vi "demandsView.vi"(10 "UserEvents in":refnum<class "UserEvents.lvclass">) -> ()   [LabVIEW 2013, in "AITDTViews.lvlib"]
uses:
  AITDTViews.lvlib
  UserEvents/UserEvents.lvclass
  CommandFactory/CommandFactory.lvclass
  UserEvents/UserEvents.lvclass/UserEvents.ctl
  Typedefs/StateSelector.ctl
  Typedefs/CommandSelector.ctl
  Typedefs/AITDTTypedefs.lvlib
  ConfigurationTestParameters/ConfigurationTestParameters.lvclass
panel:
  in  "stopTestIsTrue":bool
  in  "startTestIsTrue":bool
types:
  T1 = enum8{"Enabled", "Disabled", "Disabled and Grayed Out"}
  T2 = typedef "AITDTTypedefs.lvlib/PubDataEvents.ctl" = cluster{"State":refnum<user-event>, "ErrorCode":refnum<user-event>, "OutputData":refnum<user-event>, "InputData":refnum<user-event>, "TestStatus":refnum<user-event>, "LogPath":refnum<user-event>, "TemperatureSetpointRequest":refnum<user-event>, "TemperatureSettling":refnum<user-event>, "WaitTimeStatus":refnum<user-event>}
  T3 = typedef "AITDTTypedefs.lvlib/SubDataEvents.ctl" = cluster{"Command":refnum<user-event>}
  T4 = cluster{"Event Registration Refnum":refnum<event-registration>}
  T5 = typedef "AITDTTypedefs.lvlib/StateSelector.ctl" = enum16{"AwaitingSetpointAcknowledgmentState", "EndingCycleState", "FaultState", "OffState", "PausingState", "RequestingNewSetpointState", "SamplingState", "SettlingState", "SoakingState", "StabilizingState", "StandbyState", "StoppedState", "TransitioningTemperatureState"}
  T6 = typedef "AITDTTypedefs.lvlib/CommandSelector.ctl" = enum16{"ClearError", "ConfirmSetpointApplied", "Exit", "StandBy", "Start", "StartTest", "StopTest", "Update"}
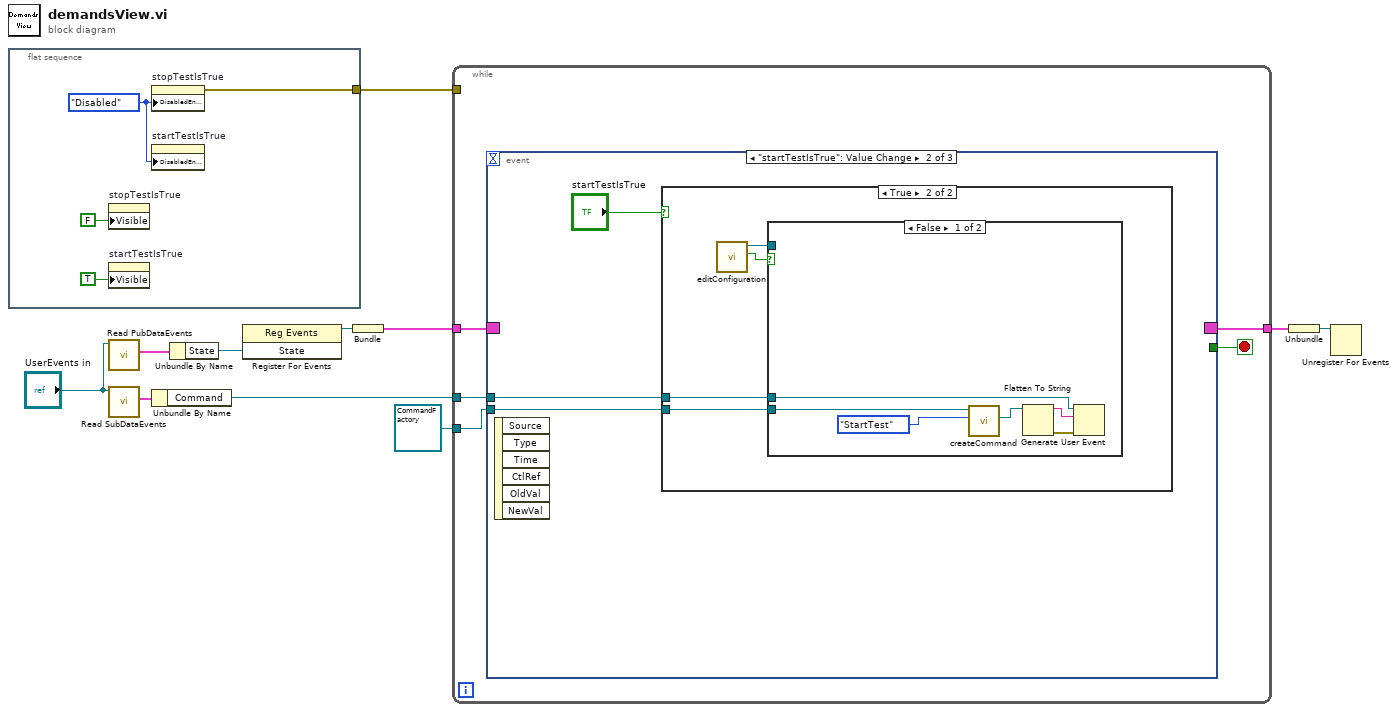
[diagram p0: block diagram]
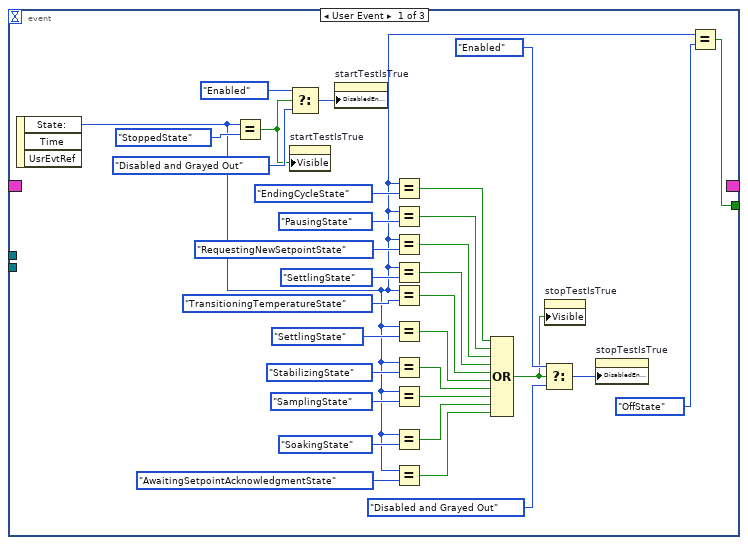
[diagram p2: hidden frame]
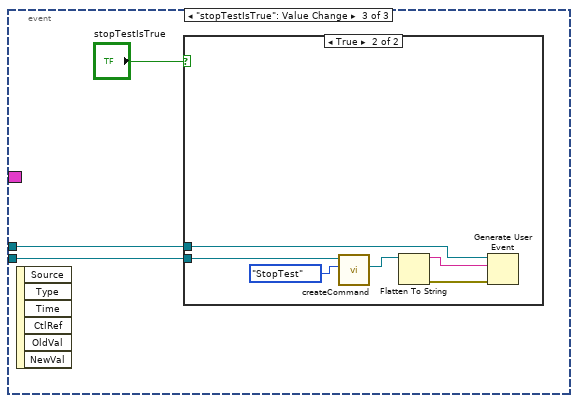
[diagram p5: hidden frame]
diagram:
  n1 = flat-sequence {
    tunnel: [w13] -> w1
    frame #0 {
      w15 = T1."Disabled" ("Disabled")
      n2 = property on="stopTestIsTrue" class="Bool"("Visible"=FALSE) -> ()  [unwired: 2 in, 2 out]
      n3 = property on="startTestIsTrue" class="Bool"("Visible"=TRUE) -> ()  [unwired: 2 in, 2 out]
      n4 = property on="stopTestIsTrue" class="Bool"("DisabledEnum"=w15) -> (error out=w13:errorcluster)  [unwired: 2 in, 1 out]
      n5 = property on="startTestIsTrue" class="Bool"("DisabledEnum"=w15) -> ()  [unwired: 2 in, 2 out]
    }
  }
  n6 = call "Read PubDataEvents.vi"("UserEvents in"="UserEvents in") -> ("PubDataEvents"=w8:T2)  [unwired: 9 in, 1 out]
  n7 = call "Read SubDataEvents.vi"("UserEvents in"="UserEvents in") -> ("SubDataEvents"=w9:T3)  [unwired: 9 in, 1 out]
  n8 = Unbundle By Name(w9) -> ("Command"=w6:refnum<user-event>)
  n9 = Unbundle By Name(w8) -> ("State"=w10:refnum<user-event>)
  n10 = register-events(w10) -> (reference out=w11:refnum<event-registration>)  [unwired: 2 in, 1 out]
  n11 = Bundle("Event Registration Refnum"=w11) -> (w7:T4)  [unwired: 1 in]
  n12 = while {
    tunnel: w7 -> [w20]
    tunnel: w6 -> [w19]
    tunnel: [w18] -> w5
    tunnel: refnum<class "CommandFactory.lvclass"> refnum ("CommandFactory.lvclass") -> [w16]
    tunnel: w1 -> [_]
    stop <- w17 stop-if-true
    n13 = event shown="[1] \"startTestIsTrue\": Value Change" {
      selector: w20 -> [_ _ _]
      dyn-events: [_ _ _] -> w18
      timeout: _ -> [_ _ _]
      tunnel: w19 -> [_ w53 w68]
      tunnel: [w50 _ _] -> w17
      tunnel: w16 -> [_ w54 w67]
      event User Event {
        n14 = event-data() -> ("State:"=w22:T5)  [unwired: 1 in, 2 out]
        n15 = Equal?(x=w22, y=StateSelector."StoppedState") -> (x = y?=w43:bool)
        n16 = Select(t=T1."Enabled" ("Disabled"), s=w43, f=T1."Disabled and Grayed Out" ("Disabled")) -> (s? t:f=w45:T1)
        n17 = property on="startTestIsTrue" class="Bool"("Visible"=w43) -> ()  [unwired: 2 in, 2 out]
        n18 = property on="startTestIsTrue" class="Bool"("DisabledEnum"=w45) -> ()  [unwired: 2 in, 2 out]
        n19 = Equal?(x=w22, y=StateSelector."EndingCycleState") -> (x = y?=w37:bool)
        n20 = Equal?(x=w22, y=StateSelector."PausingState") -> (x = y?=w36:bool)
        n21 = Equal?(x=w22, y=StateSelector."RequestingNewSetpointState") -> (x = y?=w32:bool)
        n22 = Equal?(x=w22, y=StateSelector."SettlingState") -> (x = y?=w35:bool)
        n23 = Equal?(x=w22, y=StateSelector."TransitioningTemperatureState") -> (x = y?=w34:bool)
        n24 = Equal?(x=w22, y=StateSelector."SettlingState") -> (x = y?=w28:bool)
        n25 = Equal?(x=w22, y=StateSelector."StabilizingState") -> (x = y?=w27:bool)
        n26 = Equal?(x=w22, y=StateSelector."SamplingState") -> (x = y?=w26:bool)
        n27 = Equal?(x=w22, y=StateSelector."SoakingState") -> (x = y?=w24:bool)
        n28 = Equal?(x=w22, y=StateSelector."AwaitingSetpointAcknowledgmentState") -> (x = y?=w21:bool)
        n29 = Compound Arithmetic op=OR(w37, w36, w32, w35, w34, w28, w27, w26, w24, w21) -> (w33:bool)
        n30 = Select(t=T1."Enabled" ("Disabled"), s=w33, f=T1."Disabled and Grayed Out" ("Disabled")) -> (s? t:f=w44:T1)
        n31 = property on="stopTestIsTrue" class="Bool"("Visible"=w33) -> ()  [unwired: 2 in, 2 out]
        n32 = property on="stopTestIsTrue" class="Bool"("DisabledEnum"=w44) -> ()  [unwired: 2 in, 2 out]
        n33 = Equal?(x=w22, y=StateSelector."OffState") -> (x = y?=w50:bool)
      }
      event "startTestIsTrue": Value Change {
        n34 = event-data() -> ()  [unwired: 1 in, 6 out]
        n35 = case shown="True" "startTestIsTrue" {
          tunnel: w54 -> [_ w59]
          tunnel: w53 -> [_ w58]
          frame False {
          }
          frame True {
            n36 = call "editConfiguration.vi"() -> ("cancelIsTrue out"=w56:bool, "ConfigurationThisComponent out"=w57:refnum<class "ConfigurationTestParameters.lvclass">)  [unwired: 9 in, 1 out]
            n37 = case shown="False" w56 {
              tunnel: w59 -> [w65 _]
              tunnel: w58 -> [w61 _]
              tunnel: w57 -> [_ _]
              frame False {
                n38 = call-dynamic "createCommand.vi"("Command"=CommandSelector."StartTest", "CommandFactory in"=w65) -> ("command"=w60:refnum<class "Command.lvclass">)  [unwired: 7 in, 2 out]
                n39 = Flatten To String(anything=w60) -> (data string=w62:string, error out=w63:errorcluster)  [unwired: 3 in, 1 out]
                n40 = Generate User Event(user event=w61, event data cluster=w62, error in=w63) -> ()  [unwired: 1 in, 2 out]
              }
              frame True {
              }
            }
          }
        }
      }
      event "stopTestIsTrue": Value Change {
        n41 = event-data() -> ()  [unwired: 1 in, 6 out]
        n42 = case shown="True" "stopTestIsTrue" {
          tunnel: w67 -> [_ w74]
          tunnel: w68 -> [_ w70]
          frame False {
          }
          frame True {
            n43 = call-dynamic "createCommand.vi"("Command"=CommandSelector."StopTest", "CommandFactory in"=w74) -> ("command"=w69:refnum<class "Command.lvclass">)  [unwired: 7 in, 2 out]
            n44 = Flatten To String(anything=w69) -> (data string=w71:string, error out=w72:errorcluster)  [unwired: 3 in, 1 out]
            n45 = Generate User Event(user event=w70, event data cluster=w71, error in=w72) -> ()  [unwired: 1 in, 2 out]
          }
        }
      }
    }
  }
  n46 = Unbundle(w5) -> ("Event Registration Refnum"=w4:refnum<event-registration>)
  n47 = Unregister For Events(event registration refnum=w4) -> ()  [unwired: 1 in, 1 out]
